vi "GetAlarm.vi"(8 "alarm":i32(ring)=1 items=["Latest"=1, "SecondLatest"=2, "ThirdLatest"=3, "FourthLatest"=4], 9 "HighSpeedEServer":refnum<k24>, 11 "error in (no error)":errorcluster) -> (0 "Type":i32, 1 "OccurringTime":string, 2 "Text":string, 3 "error out":errorcluster)   [LabVIEW 2013, in "UnderAutomation.Yaskawa.lvlib"]
uses:
  UnderAutomation.Yaskawa.lvlib
  C:/Users/fg/Documents/Yaskawa.vi/LabVIEW_2024/UnderAutomation.Yaskawa/lib/UnderAutomation.Yaskawa.dll
  LabVIEW_2024/UnderAutomation.Yaskawa/lib/UnderAutomation.Yaskawa.dll
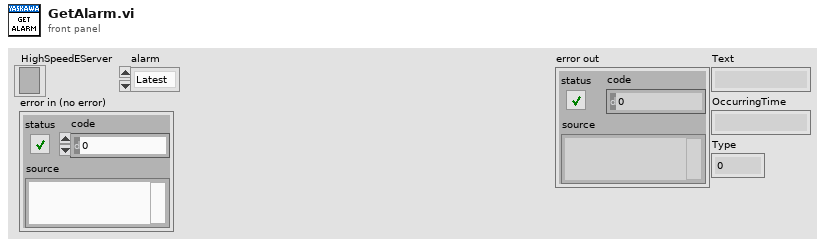
[diagram p1: front panel]
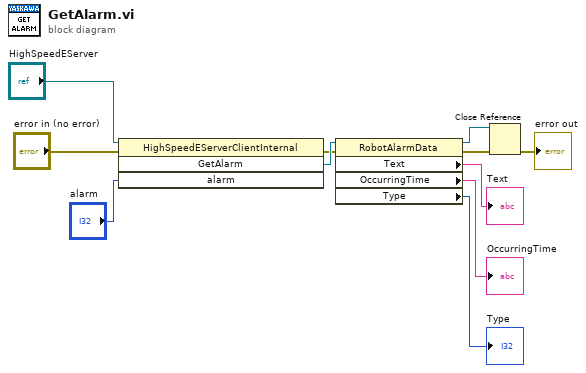
[diagram p0: block diagram]
diagram:
  n1 = invoke class="HighSpeedEServerClientInternal" method="GetAlarm"(reference="HighSpeedEServer", error in="error in (no error)", "alarm"="alarm") -> (error out=w7:errorcluster, "GetAlarm"=w8:refnum<k24>)  [unwired: 1 in, 2 out]
  n2 = property class="RobotAlarmData"(reference=w8, error in=w7) -> (reference out=w1:refnum<k24>, error out=w3:errorcluster, "Text"=→"Text":string, "OccurringTime"=→"OccurringTime":string, "Type"=→"Type":i32)
  n3 = Close Reference(reference=w1, error in (no error)=w3) -> (error out=→"error out":errorcluster)
